vi "Main.vi"() -> ()   [LabVIEW 2012]
uses:
  file_action_enum.ctl
  <vilib>/Utility/file.llb/Read From Spreadsheet File (string).vi
  <vilib>/Utility/file.llb/Write To Spreadsheet File (string).vi
panel:
  out "counter 2":i32
  in  "choice":T1=enum."convert 16-bit tiff"
  out "Slide":dbl(slide) scale=0.0..1.0
  out "counter":i32
  out "filesmoved log path":path
  out "file to transfer":path
  out "error out 2":errorcluster
  out "error out":errorcluster
  in  "button:start":bool
  in  "button:stop":bool
  in  "Tab Control":enum32{"Main", "Debug"}(tab)
  in  "Source direcory":path
  in  "Destination directory":path
  in  "file age (sec.)":dbl
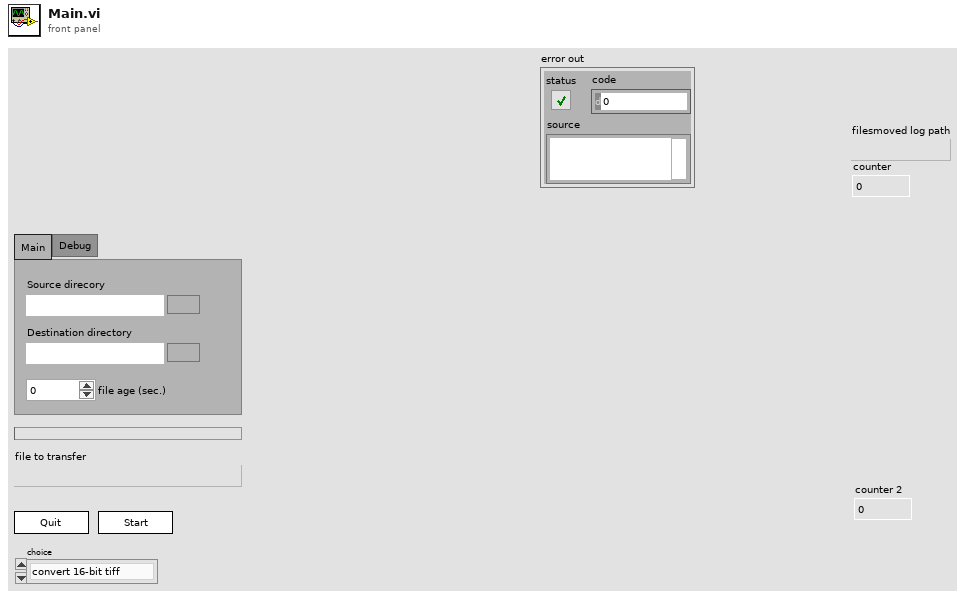
[diagram p1: front panel]
types:
  T1 = typedef "file_action_enum.ctl" = enum16{"move", "convert 16-bit tiff", "convert 8-bit tiff"}
  T2 = enum16{"open", "replace", "create", "open or create", "replace or create", "replace or create with confirmation"}
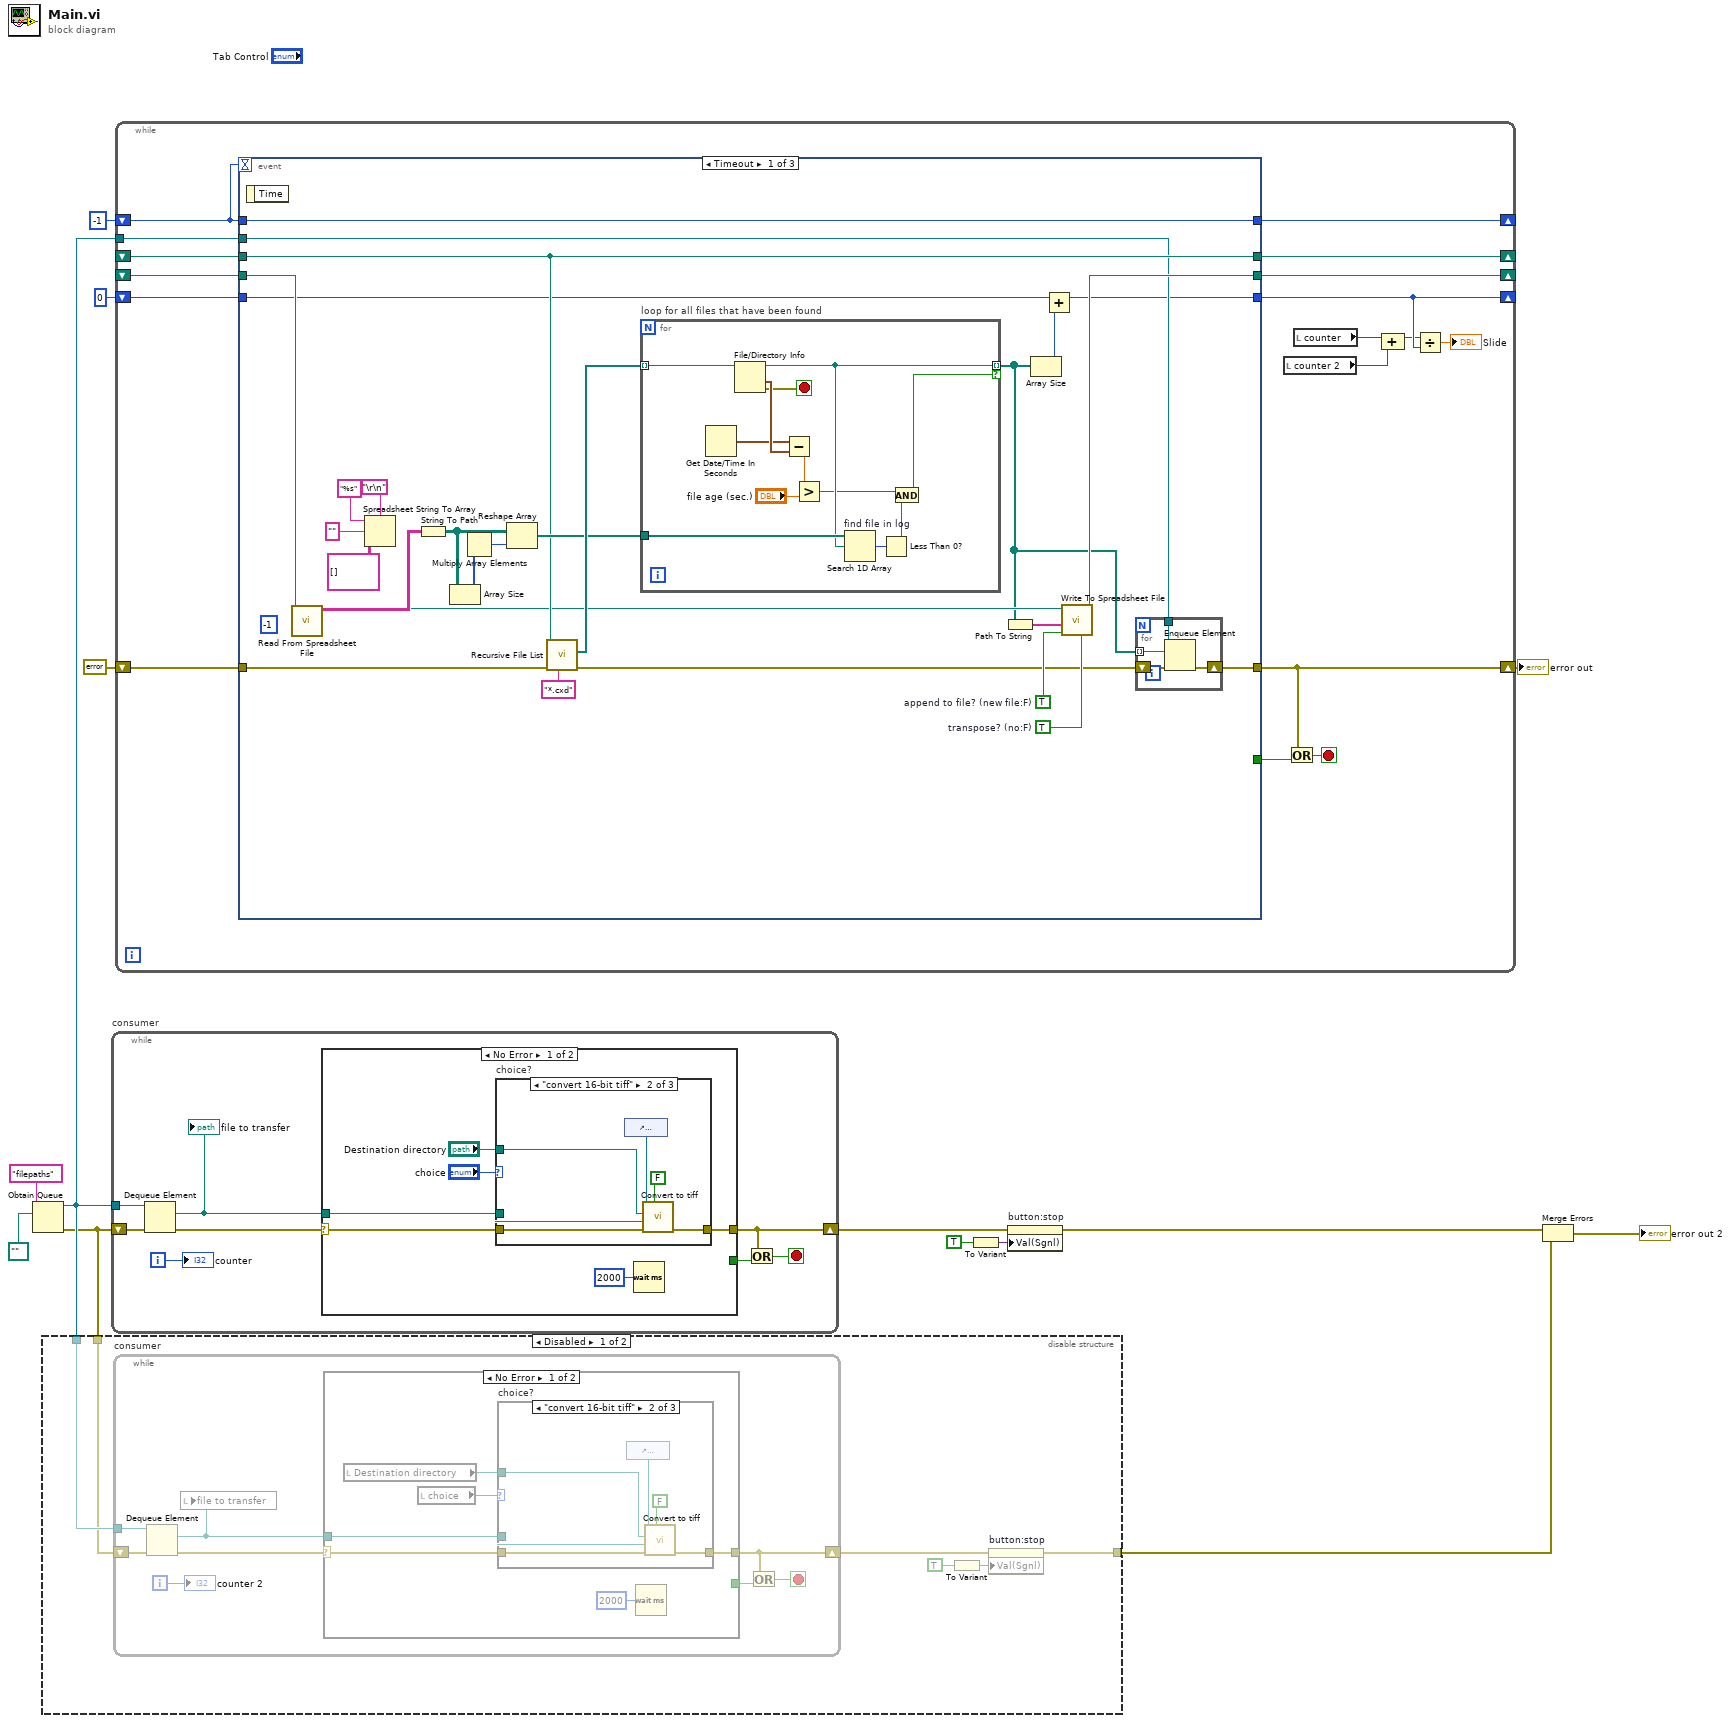
[diagram p0: block diagram]
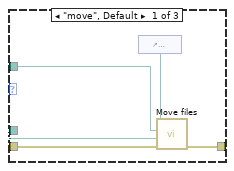
[diagram p2: hidden frame]
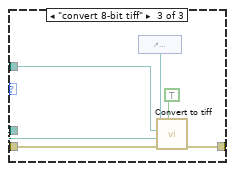
[diagram p3: hidden frame]
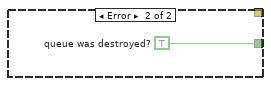
[diagram p4: hidden frame]
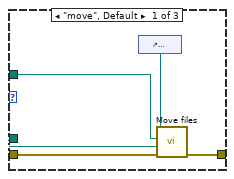
[diagram p6: hidden frame]
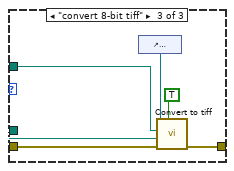
[diagram p7: hidden frame]
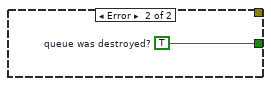
[diagram p8: hidden frame]
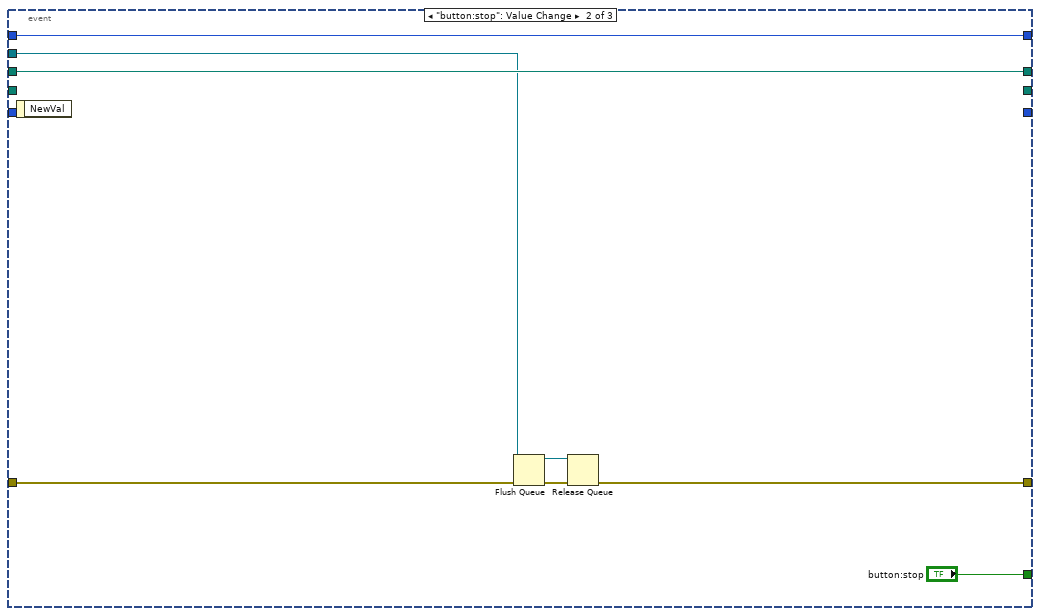
[diagram p9: hidden frame]
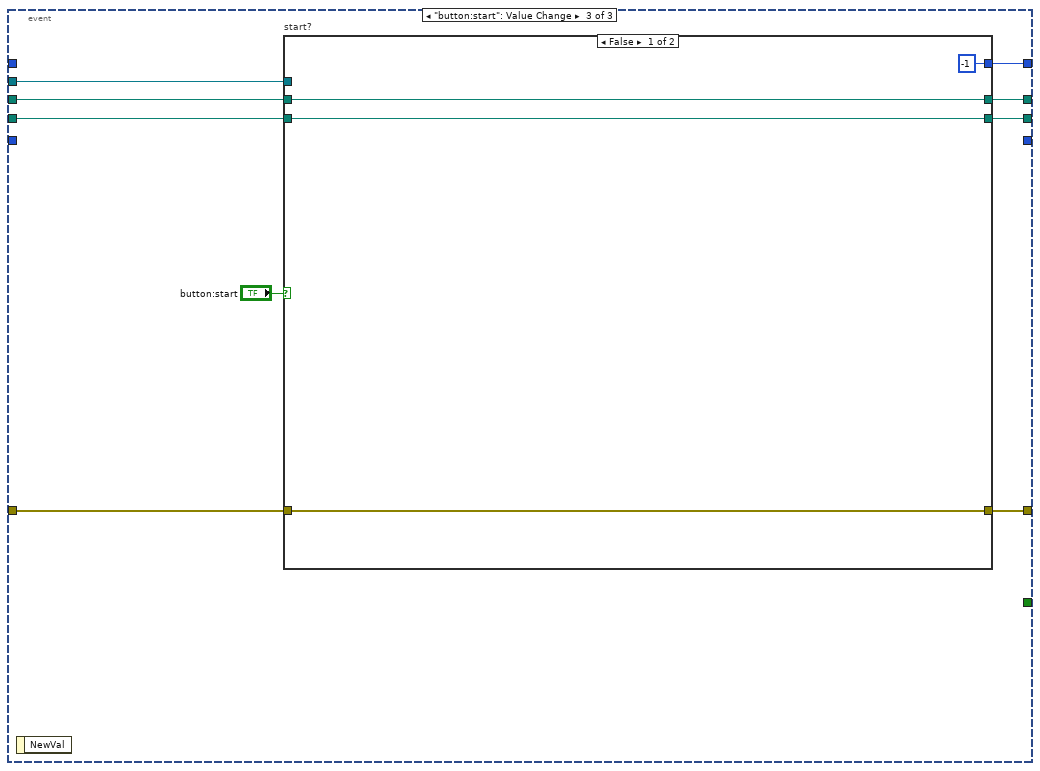
[diagram p10: hidden frame]
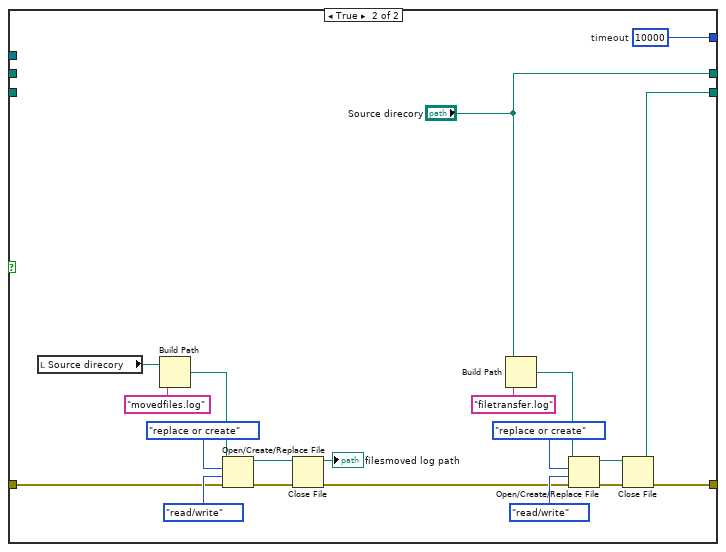
[diagram p11: hidden frame]
diagram:
  n1 = Obtain Queue(name (unnamed)="filepaths", element data type=path "" ("Destination directory")) -> (queue out=w5:refnum<queue>, error out=w4:errorcluster)  [unwired: 3 in, 1 out]
  n2 = disable-structure shown="Disabled" {
    disable-tunnel: w5 -> [w20 _]
    disable-tunnel: w4 -> [w19 _]
    disable-tunnel: [w15 _] -> w3
    frame Disabled {
      n3 = while "consumer" {
        tunnel: w20 -> [w28]
        shift-right: [w23] -> w16
        shift-left: w19 -> [w27]
        i -> [w22]
        stop <- w24 stop-if-true
        n4 = Dequeue Element(queue=w28, error in (no error)=w27) -> (element=w21:path, error out=w26:errorcluster)  [unwired: 1 in, 2 out]
        n5 = local write "file to transfer"(w21) -> ()
        n6 = case shown="No Error" w26 {
          selector: w26 -> [w33 _]
          tunnel: w21 -> [w34 _]
          tunnel: [w32 _] -> w23
          tunnel: [_ w52] -> w25
          frame No Error {
            n7 = local read "Destination directory"() -> (w29:path)
            n8 = local read "choice"() -> (w30:T1)
            n9 = case "choice?" shown="\"convert 16-bit tiff\"" w30 {
              tunnel: w34 -> [w39 w45 w51]
              tunnel: w33 -> [w38 w44 w50]
              tunnel: [w37 w43 w49] -> w32
              tunnel: w29 -> [w36 w42 w48]
              frame "move", Default {
                n10 = control-ref of="filesmoved log path"() -> (w35:refnum<vi>)
                n11 = call "Move files.vi"("error in (no error)"=w38, "source file"=w39, "Destination directory"=w36, "Path in"=w35) -> ("error out"=w37:errorcluster)  [unwired: 7 in]
              }
              frame "convert 16-bit tiff" {
                n12 = control-ref of="filesmoved log path"() -> (w41:refnum<vi>)
                n13 = call "Convert to tiff.vi"("downcast to 8-bit? (F)"=FALSE, "error in (no error)"=w44, "source file"=w45, "Destination directory"=w42, "reference to path"=w41) -> ("error out"=w43:errorcluster)  [unwired: 6 in]
              }
              frame "convert 8-bit tiff" {
                n14 = control-ref of="filesmoved log path"() -> (w47:refnum<vi>)
                n15 = call "Convert to tiff.vi"("downcast to 8-bit? (F)"=TRUE, "error in (no error)"=w50, "source file"=w51, "Destination directory"=w48, "reference to path"=w47) -> ("error out"=w49:errorcluster)  [unwired: 6 in]
              }
            }
            n16 = Wait (ms)(milliseconds to wait=u32 2000) -> ()  [unwired: 1 out]
          }
          frame Error {
            w52 = TRUE  # queue was destroyed?
          }
        }
        n17 = Or(x=w23, y=w25) -> (x .or. y?=w24:bool)
        "counter 2" <- w22
      }
      n18 = To Variant(anything=TRUE) -> (Variant=w18:variant)
      n19 = property on="button:stop" class="Bool"(error in=w16, "Val(Sgnl)"=w18) -> (error out=w15:errorcluster)  [unwired: 1 in, 1 out]
    }
    frame Enabled {
    }
  }
  n20 = while "consumer" {
    tunnel: w5 -> [w60]
    shift-right: [w54] -> w9
    shift-left: w4 -> [w59]
    i -> [w53]
    stop <- w55 stop-if-true
    n21 = Dequeue Element(queue=w60, error in (no error)=w59) -> (element=w58:path, error out=w57:errorcluster)  [unwired: 1 in, 2 out]
    "file to transfer" <- w58
    n22 = case shown="No Error" w57 {
      selector: w57 -> [w65 _]
      tunnel: w58 -> [w66 _]
      tunnel: [w64 _] -> w54
      tunnel: [_ w84] -> w56
      frame No Error {
        n23 = case "choice?" shown="\"convert 16-bit tiff\"" "choice" {
          tunnel: w66 -> [w71 w77 w83]
          tunnel: w65 -> [w70 w76 w82]
          tunnel: [w69 w75 w81] -> w64
          tunnel: "Destination directory" -> [w68 w74 w80]
          frame "move", Default {
            n24 = control-ref of="filesmoved log path"() -> (w67:refnum<vi>)
            n25 = call "Move files.vi"("error in (no error)"=w70, "source file"=w71, "Destination directory"=w68, "Path in"=w67) -> ("error out"=w69:errorcluster)  [unwired: 7 in]
          }
          frame "convert 16-bit tiff" {
            n26 = control-ref of="filesmoved log path"() -> (w73:refnum<vi>)
            n27 = call "Convert to tiff.vi"("downcast to 8-bit? (F)"=FALSE, "error in (no error)"=w76, "source file"=w77, "Destination directory"=w74, "reference to path"=w73) -> ("error out"=w75:errorcluster)  [unwired: 6 in]
          }
          frame "convert 8-bit tiff" {
            n28 = control-ref of="filesmoved log path"() -> (w79:refnum<vi>)
            n29 = call "Convert to tiff.vi"("downcast to 8-bit? (F)"=TRUE, "error in (no error)"=w82, "source file"=w83, "Destination directory"=w80, "reference to path"=w79) -> ("error out"=w81:errorcluster)  [unwired: 6 in]
          }
        }
        n30 = Wait (ms)(milliseconds to wait=u32 2000) -> ()  [unwired: 1 out]
      }
      frame Error {
        w84 = TRUE  # queue was destroyed?
      }
    }
    n31 = Or(x=w54, y=w56) -> (x .or. y?=w55:bool)
    "counter" <- w53
  }
  n32 = while {
    shift-right: [w100] -> _
    shift-left: -1 -> [w99]
    shift-right: [w98] -> _
    shift-left: _ -> [w101]
    shift-right: [w94] -> w12
    shift-left: errorcluster {"status"=FALSE, "code"=0, "source"=""} ("error out") -> [w97]
    shift-right: [w96] -> _
    shift-left: _ -> [w95]
    tunnel: w5 -> [w91]
    shift-right: [w89] -> _
    shift-left: 0 -> [w90]
    stop <- w93 stop-if-true
    n33 = event shown="[0] Timeout" {
      selector: _ -> [_ _ _]
      dyn-events: _ -> [_ _ _]
      timeout: w99 -> [_ _ _]
      tunnel: w101 -> [w121 _ w154]
      tunnel: [_ "button:stop" _] -> w92
      tunnel: [w109 w151 w161] -> w100
      tunnel: w99 -> [w109 w151 _]
      tunnel: [w113 _ w159] -> w98
      tunnel: [w106 w145 w158] -> w94
      tunnel: w97 -> [w115 w146 w157]
      tunnel: [w123 w150 w160] -> w96
      tunnel: w95 -> [w123 w150 w155]
      tunnel: w91 -> [w108 w149 w153]
      tunnel: [w103 _ _] -> w89
      tunnel: w90 -> [w102 _ _]
      event Timeout {
        w110 = TRUE  # transpose? (no:F)
        w111 = TRUE  # append to file? (new file:F)
        (unwired) -1 ("count")
        n34 = event-data() -> ()  [unwired: 1 in, 1 out]
        n35 = call-poly <vilib>:"Read From Spreadsheet File.vi"("file path (dialog if empty)"=w121) -> ("all rows"=w117:string[][], "new file path (Not A Path if cancelled)"=w114:path)  [unwired: 6 in, 3 out]
        n36 = Spreadsheet String To Array(delimiter (Tab)="\r\n", format string="%s", spreadsheet string="", array type (2D Dbl)=string[][] []) -> ()  [unwired: 1 out]
        n37 = String To Path(string=w117) -> (path=w126:path[][])
        n38 = Array Size(array=w126) -> (size(s)=w120:i32[])
        n39 = Multiply Array Elements(1:w120) -> (0:w119:i32)
        n40 = Reshape Array(w126, w119) -> (w125:path[])
        n41 = call <vilib>:"Recursive File List.vi"("pattern"="*.cxd", "error in (no error)"=w115, "Folder Path"=w123) -> ("error out"=w107:errorcluster, "All Files in Dir"=w128:path[])  [unwired: 4 in, 3 out]
        n42 = for "loop for all files that have been found" {
          tunnel: w128 -> [w144] mode=indexing
          tunnel: [w138] -> w105 mode=indexing if=w134
          tunnel: w125 -> [w139]
          stop <- w140 stop-if-true
          n43 = Get Date/Time In Seconds() -> (seconds since 1Jan1904=w142:timestamp)
          n44 = File/Directory Info(path=w144) -> (path out=w138:path, last mod=w143:timestamp, error out=w140:errorcluster)  [unwired: 1 in, 4 out]
          n45 = Subtract(x=w142, y=w143) -> (x-y=w133:dbl)
          n46 = Greater?(x=w133, y="file age (sec.)") -> (0:w136:bool)
          n47 = Search 1D Array "find file in log"(1D array=w139, element=w138) -> (index of element=w137:i32)  [unwired: 1 in]
          n48 = Less Than 0?(x=w137) -> (x < 0?=w135:bool)
          n49 = And(x=w136, y=w135) -> (x .and. y?=w134:bool)
        }
        n50 = Path To String(path=w105) -> (string=w112:string[])
        n51 = Array Size(array=w105) -> (size(s)=w104:i32)
        n52 = Add(x=w102, y=w104) -> (x+y=w103:i32)
        n53 = call-poly <vilib>:"Write To Spreadsheet File.vi"("transpose? (no:F)"=w110, "append to file? (new file:F)"=w111, "1D data"=w112, "file path (dialog if empty)"=w114) -> ("new file path (Not A Path if cancelled)"=w113:path)  [unwired: 4 in]
        n54 = for {
          tunnel: w108 -> [w132]
          tunnel: w105 -> [w129] mode=indexing
          shift-right: [w130] -> w106
          shift-left: w107 -> [w131]
          n55 = Enqueue Element(queue=w132, element=w129, error in (no error)=w131) -> (error out=w130:errorcluster)  [unwired: 1 in, 2 out]
        }
      }
      event "button:stop": Value Change {
        n56 = event-data() -> ()  [unwired: 1 in, 1 out]
        n57 = Flush Queue(queue=w149, error in (no error)=w146) -> (queue out=w148:refnum<queue>, error out=w147:errorcluster)  [unwired: 1 out]
        n58 = Release Queue(queue=w148, error in (no error)=w147) -> (error out=w145:errorcluster)  [unwired: 1 in, 2 out]
      }
      event "button:start": Value Change {
        n59 = event-data() -> ()  [unwired: 1 in, 1 out]
        n60 = case "start?" shown="False" "button:start" {
          tunnel: [-1 ("timeout") w185] -> w161
          tunnel: [w164 "Source direcory"] -> w160
          tunnel: [w163 w178] -> w159
          tunnel: [w162 w176] -> w158
          tunnel: w157 -> [w162 w167]
          tunnel: w155 -> [w164 _]
          tunnel: w154 -> [w163 _]
          tunnel: w153 -> [_ _]
          frame False {
          }
          frame True {
            w185 = 10000  # timeout
            n61 = local read "Source direcory"() -> (w175:path)
            n62 = Build Path(base path=w175, name or relative path="movedfiles.log") -> (appended path=w174:path)
            n63 = Open/Create/Replace File(file path (use dialog)=w174, error in=w167, operation (0:open)=T2."replace or create", access (0:read/write)=enum16{"read/write", "read-only", "write-only"}."read/write") -> (refnum out=w170:refnum<file>, error out=w168:errorcluster)  [unwired: 2 in, 1 out]
            n64 = Close File(refnum=w170, error in=w168) -> (path=→"filesmoved log path":path, error out=w166:errorcluster)
            n65 = Build Path(base path="Source direcory", name or relative path="filetransfer.log") -> (appended path=w184:path)
            n66 = Open/Create/Replace File(file path (use dialog)=w184, error in=w166, operation (0:open)=T2."replace or create", access (0:read/write)=enum16{"read/write", "read-only", "write-only"}."read/write") -> (refnum out=w179:refnum<file>, error out=w177:errorcluster)  [unwired: 2 in, 1 out]
            n67 = Close File(refnum=w179, error in=w177) -> (path=w178:path, error out=w176:errorcluster)
          }
        }
      }
    }
    n68 = local read "counter 2"() -> (w87:i32)
    n69 = Or(x=w94, y=w92) -> (x .or. y?=w93:bool)
    n70 = local read "counter"() -> (w86:i32)
    n71 = Compound Arithmetic op=ADD(w86, w87) -> (w85:i32)
    n72 = Divide(x=w85, y=w89) -> (x/y=→"Slide":dbl)
  }
  "error out" <- w12
  n73 = To Variant(anything=TRUE) -> (Variant=w7:variant)
  n74 = property on="button:stop" class="Bool"(error in=w9, "Val(Sgnl)"=w7) -> (error out=w2:errorcluster)  [unwired: 1 in, 1 out]
  n75 = Merge Errors(w2, w3) -> (→"error out 2":errorcluster)
